vi "Test Test Pass if Expected Multiple API Call Made Reverse Order.vi"(8 "error in (no error)":errorcluster, 11 "Test Case In":refnum<class "One Expectation Test.lvclass">) -> (0 "error out":errorcluster, 3 "Test Case Out":refnum<class "One Expectation Test.lvclass">)   [LabVIEW 2020, in "One Expectation Test.lvclass"]
uses:
  One Expectation Test.lvclass
  C:/Program Files (x86)/National Instruments/LabVIEW 2020/vi.lib/Astemes/LUnit/Test Case.lvclass
  Test Doubles/Test Interface Responsive Mock/Test Interface Mock.lvclass
  C:/git/astemes-lmock/source/Framework/Mock/Mock.lvclass
  source/Expectations/One/One Identical Inputs.vi
  source/Expectations/One/One.lvlib
  Expectation Test/Expectation Test.lvclass
  C:/git/astemes-lmock/tests/Test Doubles/Test Interface Responsive Mock/Test Interface Mock.lvclass
  C:/git/astemes-lmock/tests/Test Doubles/Test Interface/Test Interface.lvclass
  source/Framework/LMock API.lvlib
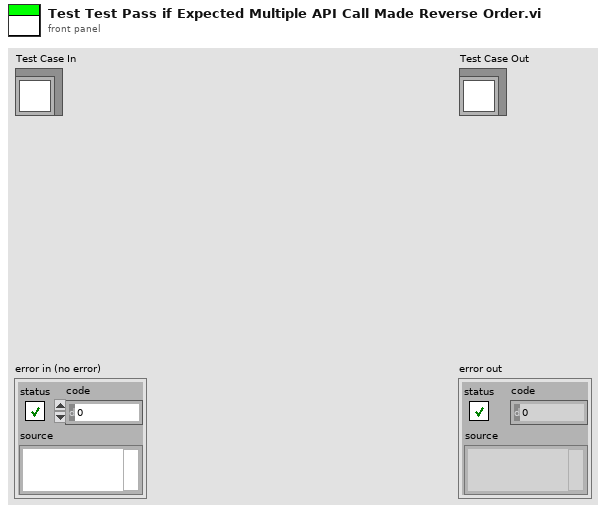
[diagram p1: front panel]
types:
  T1 = enum16{"", "Passed", "Failed", "Error", "Skipped", "Setup Error", "Broken", "Teardown Error"}
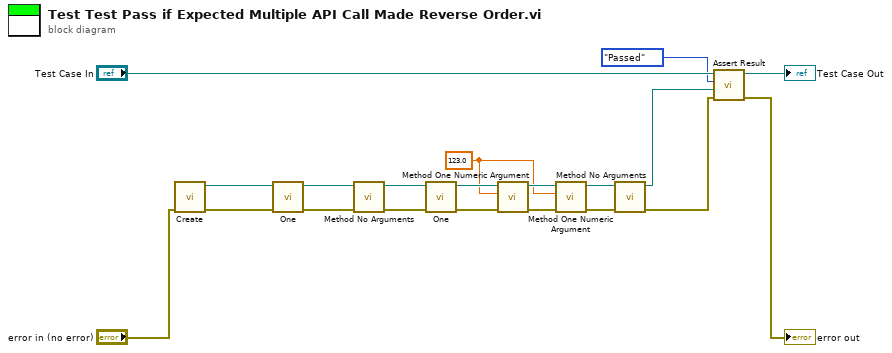
[diagram p0: block diagram]
diagram:
  w2 = 123.0 ("Numeric")
  n1 = call "Create.vi"("error in (no error)"="error in (no error)") -> ("error out"=w19:errorcluster, "Test Interface Mock Out"=w20:refnum<class "Test Interface Mock.lvclass">)  [unwired: 9 in]
  n2 = call-poly "One.vi"("error in (no error)"=w19, "Mock in"=w20) -> ("error out"=w17:errorcluster, "Mock out"=w18:refnum<class "Test Interface Mock.lvclass">)  [unwired: 8 in]
  n3 = call-dynamic "Method No Arguments.vi"("error in (no error)"=w17, "Mock In"=w18) -> ("error out"=w16:errorcluster, "Mock Out"=w9:refnum<class "Test Interface Mock.lvclass">)  [unwired: 8 in]
  n4 = call-poly "One.vi"("error in (no error)"=w16, "Mock in"=w9) -> ("error out"=w10:errorcluster, "Mock out"=w8:refnum<class "Test Interface Mock.lvclass">)  [unwired: 8 in]
  n5 = call-dynamic "Method One Numeric Argument.vi"("error in (no error)"=w10, "Numeric"=w2, "Test Interface Mock In"=w8) -> ("error out"=w6:errorcluster, "Test Interface Mock Out"=w4:refnum<class "Test Interface Mock.lvclass">)  [unwired: 7 in]
  n6 = call-dynamic "Method One Numeric Argument.vi"("error in (no error)"=w6, "Numeric"=w2, "Test Interface Mock In"=w4) -> ("error out"=w5:errorcluster, "Test Interface Mock Out"=w3:refnum<class "Test Interface Mock.lvclass">)  [unwired: 7 in]
  n7 = call-dynamic "Method No Arguments.vi"("error in (no error)"=w5, "Mock In"=w3) -> ("error out"=w7:errorcluster, "Mock Out"=w1:refnum<class "Test Interface Mock.lvclass">)  [unwired: 8 in]
  n8 = call "Assert Result.vi"("error in (no error)"=w7, "Mock"=w1, "Status"=T1."Passed", "LUnit Test Case In"="Test Case In") -> ("error out"=→"error out":errorcluster, "LUnit Test Case Out"=→"Test Case Out":refnum<class "One Expectation Test.lvclass">)  [unwired: 6 in]
